vi "Facade 1.vi"(0 "Data In":T4, 2 "Display State In":T2, 3 "Container State":T3) -> (6 "Data Out":T4, 7 "Display State Out":T2, 8 "Action":T1)   [LabVIEW 2011, in "ChangeColorBtn.xctl"]
uses:
  ChangeColorBtn.xctl
  Data 1.ctl
  <vilib>/_xctls/Container State.ctl
  State 1.ctl
  <vilib>/_xctls/Action.ctl
  <vilib>/_xctls/XControlSupport.lvlib
panel:
  in  "确定按钮":bool
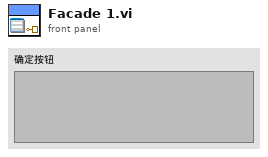
[diagram p1: front panel]
types:
  T1 = typedef "XControlSupport.lvlib/Action.ctl" = cluster{"Data Changed?":bool, "State Changed?":bool, "Action Name":string}
  T2 = typedef "ChangeColorBtn.xctl/State 1.ctl" = cluster{"鼠标进入标题":string, "鼠标离开标题":string, "鼠标进入颜色":cluster{"Color Box":u32, "Color Box 2":u32}[], "鼠标离开颜色":cluster{"Color Box":u32, "Color Box 2":u32}[]}
  T3 = typedef "XControlSupport.lvlib/Container State.ctl" = cluster{"Indicator?":bool, "Run Mode?":bool, " Refnum":refnum<vi>}
  T4 = typedef "ChangeColorBtn.xctl/Data 1.ctl" = bool
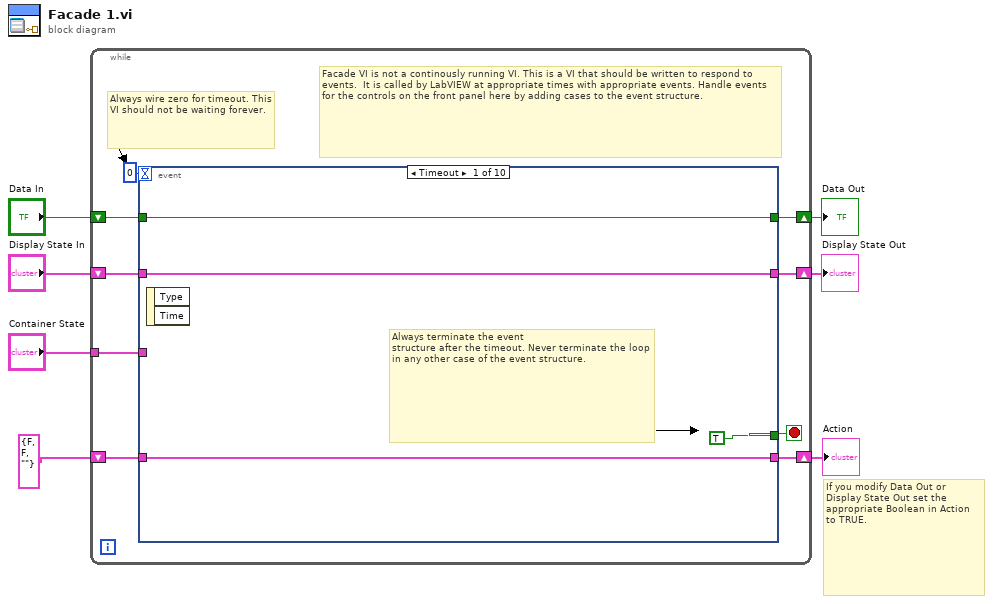
[diagram p0: block diagram]
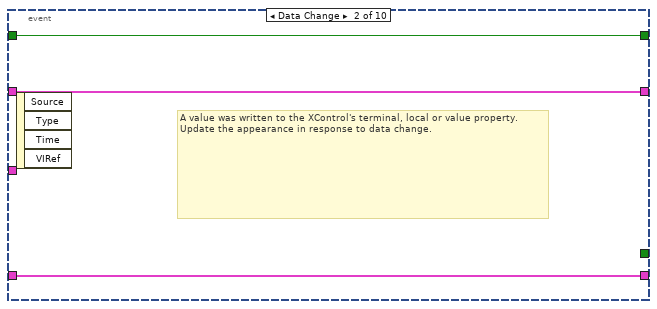
[diagram p2: hidden frame]
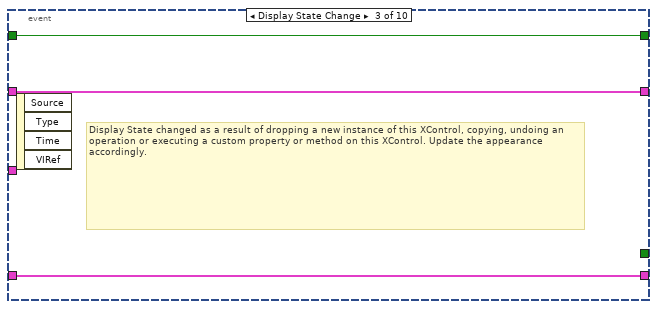
[diagram p3: hidden frame]
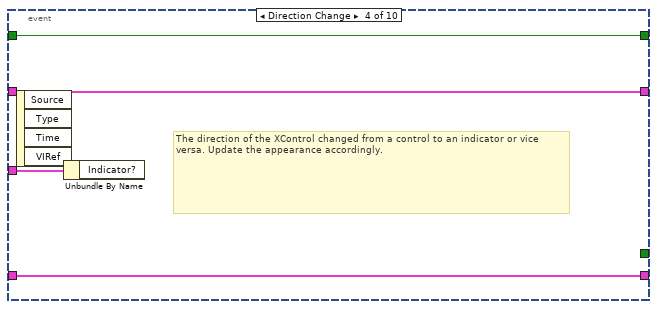
[diagram p4: hidden frame]
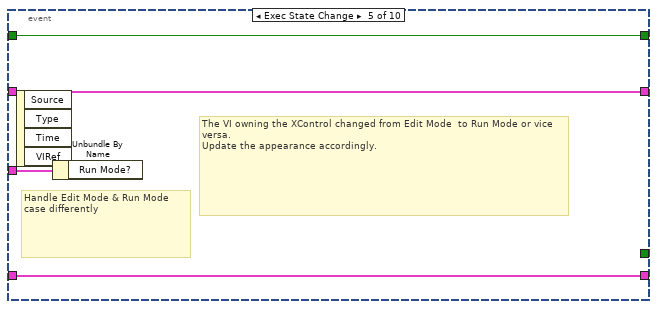
[diagram p5: hidden frame]
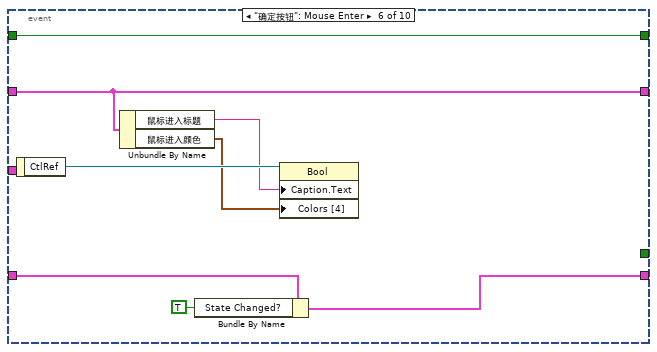
[diagram p6: hidden frame]
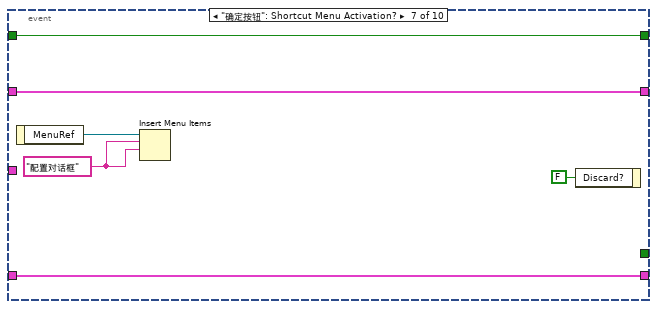
[diagram p7: hidden frame]
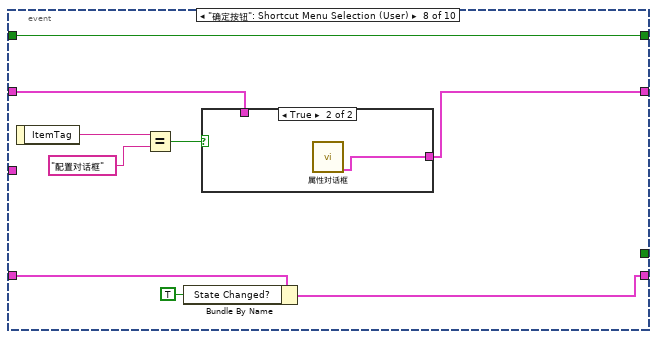
[diagram p8: hidden frame]
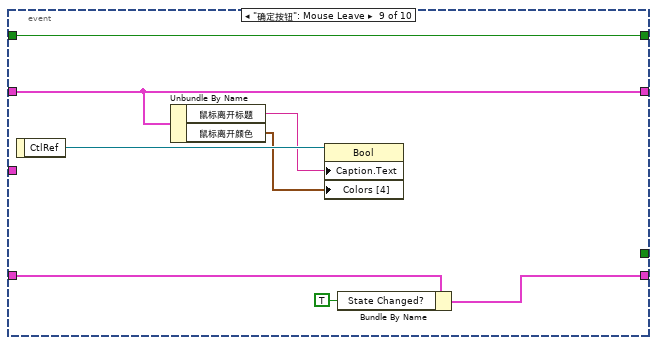
[diagram p10: hidden frame]
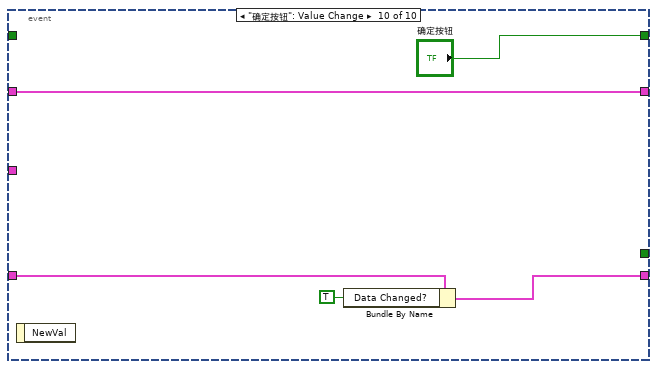
[diagram p11: hidden frame]
diagram:
  # "If you modify Data Out or\nDisplay State Out set the\nappropriate Boolean in Action\nto TRUE."
  n1 = while {
    shift-right: [w15] -> w4
    shift-left: "Display State In" -> [w16]
    tunnel: "Container State" -> [w12]
    shift-right: [w10] -> w7
    shift-left: "Data In" -> [w11]
    shift-right: [w8] -> w2
    shift-left: T1 {"Data Changed?"=FALSE, "State Changed?"=FALSE, "Action Name"=""} ("Action") -> [w9]
    stop <- w14 stop-if-true
    # "Facade VI is not a continously running VI. This is a VI that should be written to respond to events.  It is called by LabVIEW at appropriate times with appropriate events. Handle events for the controls on the front panel here by adding cases to the event structure."
    # "Always wire zero for timeout. This\nVI should not be waiting forever."
    n2 = event shown="[0] Timeout" {
      selector: _ -> [_ _ _ _ _ _ _ _ _ _]
      dyn-events: _ -> [_ _ _ _ _ _ _ _ _ _]
      timeout: 0 -> [_ _ _ _ _ _ _ _ _ _]
      tunnel: w16 -> [w18 w22 w26 w29 w33 w38 w47 w50 w66 w71]
      tunnel: [w18 w22 w26 w29 w33 w38 w47 w49 w66 w71] -> w15
      tunnel: [TRUE _ _ _ _ _ _ _ _ _] -> w14
      tunnel: w12 -> [_ _ _ w30 w34 _ _ _ _ _]
      tunnel: w11 -> [w17 w23 w25 w28 w32 w42 w48 w57 w67 _]
      tunnel: [w17 w23 w25 w28 w32 w42 w48 w57 w67 "确定按钮"] -> w10
      tunnel: [w19 w21 w24 w27 w31 w40 w46 w55 w61 w69] -> w8
      tunnel: w9 -> [w19 w21 w24 w27 w31 w41 w46 w56 w62 w70]
      event Timeout {
        # "Always terminate the event\nstructure after the timeout. Never terminate the loop in any other case of the event structure."
        n3 = event-data() -> ()  [unwired: 1 in, 2 out]
      }
      event Data Change {
        # "A value was written to the XControl's terminal, local or value property.\nUpdate the appearance in response to data change."
        n4 = event-data() -> ()  [unwired: 1 in, 4 out]
      }
      event Display State Change {
        # "Display State changed as a result of dropping a new instance of this XControl, copying, undoing an operation or executing a custom property or method on this XControl. Update the appearance accordingly."
        n5 = event-data() -> ()  [unwired: 1 in, 4 out]
      }
      event Direction Change {
        # "The direction of the XControl changed from a control to an indicator or vice versa. Update the appearance accordingly."
        n6 = event-data() -> ()  [unwired: 1 in, 4 out]
        n7 = Unbundle By Name(w30) -> ()  [unwired: 1 out]
      }
      event Exec State Change {
        # "The VI owning the XControl changed from Edit Mode  to Run Mode or vice versa.\nUpdate the appearance accordingly."
        # "Handle Edit Mode & Run Mode\ncase differently"
        n8 = event-data() -> ()  [unwired: 1 in, 4 out]
        n9 = Unbundle By Name(w34) -> ()  [unwired: 1 out]
      }
      event "确定按钮": Mouse Enter {
        n10 = event-data() -> ("CtlRef"=w37:refnum<vi>)  [unwired: 1 in]
        n11 = Unbundle By Name(w38) -> ("鼠标进入标题"=w36:string, "鼠标进入颜色"=w35:cluster{"Color Box":u32, "Color Box 2":u32}[])
        n12 = Bundle By Name(cluster=w41, "State Changed?"=TRUE ("Data Changed?")) -> (w40:T1)
        n13 = property class="Bool"(reference=w37, "Caption.Text"=w36, "Colors [4]"=w35) -> ()  [unwired: 1 in, 2 out]
      }
      event "确定按钮": Shortcut Menu Activation? {
        w43 = "配置对话框"
        n14 = event-data() -> ("MenuRef"=w44:refnum<k9>)  [unwired: 1 in]
        n15 = Insert Menu Items(7:w43, 8:w43, 9:w44) -> ()  [unwired: 3 in, 3 out]
        n16 = event-data("Discard?"=FALSE) -> ()  [unwired: 1 in, 1 out]
      }
      event "确定按钮": Shortcut Menu Selection (User) {
        n17 = event-data() -> ("ItemTag"=w53:string)  [unwired: 1 in]
        n18 = Equal?(x=w53, y="配置对话框") -> (x = y?=w51:bool)
        n19 = Bundle By Name(cluster=w56, "State Changed?"=TRUE ("Data Changed?")) -> (w55:T1)
        n20 = case shown="True" w51 {
          tunnel: w50 -> [w58 _]
          tunnel: [w58 w59] -> w49
          frame False {
          }
          frame True {
            n21 = call "属性对话框.vi"() -> ("State"=w59:T2)  [unwired: 11 in]
          }
        }
      }
      event "确定按钮": Mouse Leave {
        n22 = event-data() -> ("CtlRef"=w65:refnum<vi>)  [unwired: 1 in]
        n23 = Unbundle By Name(w66) -> ("鼠标离开标题"=w63:string, "鼠标离开颜色"=w64:cluster{"Color Box":u32, "Color Box 2":u32}[])
        n24 = property class="Bool"(reference=w65, "Caption.Text"=w63, "Colors [4]"=w64) -> ()  [unwired: 1 in, 2 out]
        n25 = Bundle By Name(cluster=w62, "State Changed?"=TRUE ("Data Changed?")) -> (w61:T1)
      }
      event "确定按钮": Value Change {
        n26 = event-data() -> ()  [unwired: 1 in, 1 out]
        n27 = Bundle By Name(cluster=w70, "Data Changed?"=TRUE) -> (w69:T1)
      }
    }
  }
  "Display State Out" <- w4
  "Data Out" <- w7
  "Action" <- w2
